vi "TEST - Parse String with TDs.vi"(8 "error in (no error)":errorcluster) -> (0 "error out":errorcluster, 2 "pass":bool)   [LabVIEW 2020, in "test_openg_array.lvlib"]
uses:
  test_openg_array.lvlib
  <userlib>/_OpenG.lib/error/error.llb/openg_error.lvlib
  source/library/openg_variant.lvlib
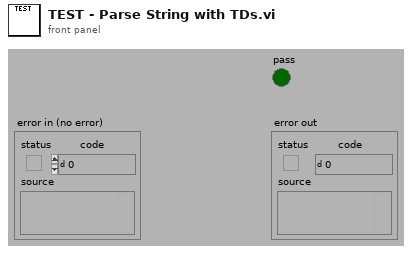
[diagram p1: front panel]
types:
  T1 = typedef "openg_variant.lvlib/Type Descriptor.ctl" = i16[]
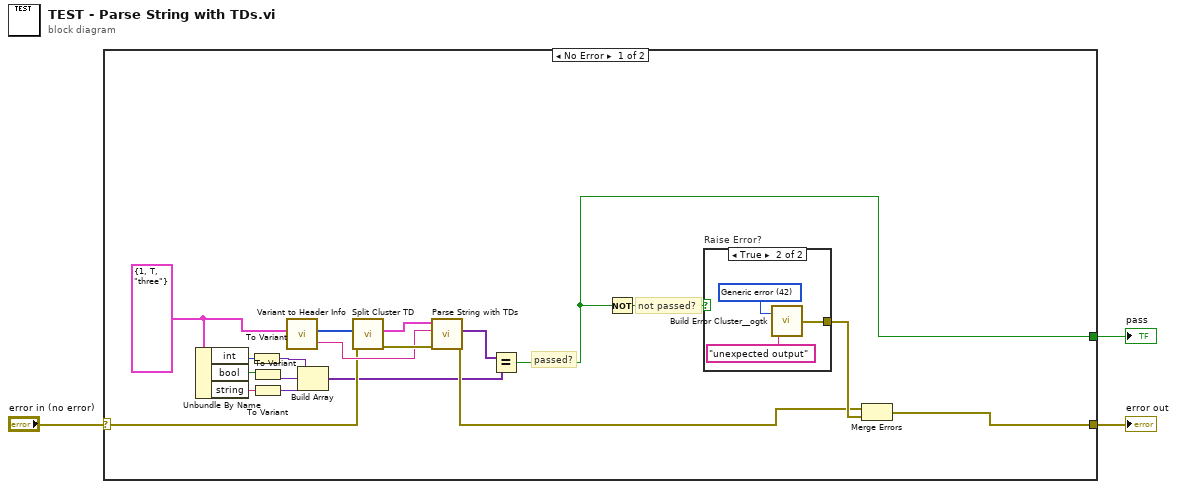
[diagram p0: block diagram]
diagram:
  n1 = case shown="No Error" "error in (no error)" {
    selector: "error in (no error)" -> [w14 w26]
    tunnel: [w4 _] -> w3
    tunnel: [w22 w26] -> w1
    frame No Error {
      w13 = cluster{"int":i32, "bool":bool, "string":string} {"int"=1, "bool"=TRUE, "string"="three"}
      # "not passed?"
      # "passed?"
      n2 = Unbundle By Name(w13) -> ("int"=w12:i32, "bool"=w11:bool, "string"=w10:string)
      n3 = To Variant(anything=w12) -> (Variant=w9:variant)
      n4 = To Variant(anything=w11) -> (Variant=w8:variant)
      n5 = To Variant(anything=w10) -> (Variant=w7:variant)
      n6 = call "Variant to Header Info.vi"("Variant"=w13) -> ("Type Descriptor"=w16:T1, "data string"=w17:string)  [unwired: 3 in, 1 out]
      n7 = Build Array(w9, w8, w7) -> (w5:variant[])
      n8 = call "Split Cluster TD.vi"("error in (no error)"=w14, "Type Descriptor"=w16) -> ("error out"=w18:errorcluster, "Type Descriptors"=w19:cluster{"Type Descriptor":T1}[])  [unwired: 8 in]
      n9 = call "Parse String with TDs.vi"("error in (no error)"=w18, "Data string"=w17, "Type Descriptors"=w19) -> ("error out"=w15:errorcluster, "Array of VData"=w6:variant[])  [unwired: 6 in, 1 out]
      n10 = Equal?(x=w6, y=w5) -> (x = y?=w4:bool)
      n11 = Not(x=w4) -> (.not. x?=w20:bool)
      n12 = case "Raise Error?" shown="True" w20 {
        tunnel: [_ w23] -> w21
        frame False {
        }
        frame True {
          w24 = 42 items=["No error", "Argument error", "Memory is full", "Out of zone", "End of file", "File already open", "Generic file I/O error", "File not found", "File permission error", "Disk is full", "Duplicate path", "Too many files open", "System feature not enabled", "Resource file not found", "Cannot add resource", "Resource not found", "Image not found", "Image memory error", "Pen does not exist", "Config type invalid", "Config token not found", "Config parse error", "Config memory error", "Bad external code format", "Bad external code offset", "External code not present", "Null window", "Destroy window error", "Null menu", "Print aborted", "Bad print record", "Print driver error", "Windows error during printing", "Memory error during printing", "Print dialog error", "Generic print error", "Invalid device refnum", "Device not found", "Device parameter error", "Device unit error", "Cannot open device", "Device call aborted", "Generic error", "Cancelled by user", "Object ID too low", "Object ID too high", "Object not in heap", "Unknown heap", "Unknown object (invalid DefProc)", "Unknown object (DefProc not in table)", "Message out of range", "Invalid (null) method", "Unknown message", "Manager call not supported", "Bad address", "Network operation in progress", "Network operation timed out", "Connection is busy", "Network attribute not supported", "Network error", "Address in use", "System out of memory", "Connection aborted", "Connection refused", "Not connected", "Already connected", "Connection closed", "Initialization error (interapplication manager)", "Bad occurrence", "Wait on unbound occurrence handler", "Occurrence queue overflow", "Datalog type conflict", "Unused", "Unrecognized type (interapplication manager)", "Memory corrupt", "Failed to make temporary DLL", "Old CIN version", "Drag socket not found", "Failed to load drop-object", "Failed to register OLE object", "Failed to release OLE object", "Format specifier type mismatch", "Unknown format specifier", "Too few format specifiers", "Too many format specifiers", "Scan failed", "Newer CIN version", "Error converting to variant", "Runtime menu error", "Password tampered", "Variant attribute not found", "Incompatible variant data type", "Event data is not available", "Event Store is not present", "Occurrence is not found", "Event Queue is not created", "Event info is not available", "Refnum passed is NULL", "Error retrieving Class GUID", "Error retrieving CoClass GUID", "Error retrieving TypeLib GUID.", "Bad built application magic bytes.", "Specific driver is different from the specific driver associated with the Logical Name.", "There is no session opened to the class driver.", "Max Error", "MAX - Error with config objects", "MAX - Error loading configuration", "MAX - Group not supported"]
          n13 = call <userlib>:"Build Error Cluster__ogtk.vi"("String to Prepend to source (\"\")"="unexpected output" ("String to Prepend to source (\"\")"), "code"=w24) -> ("error out"=w23:errorcluster)
        }
      }
      n14 = Merge Errors(w15, w21) -> (w22:errorcluster)
    }
    frame Error {
    }
  }
  "pass" <- w3
  "error out" <- w1
